vi "Distance + Height to Angle + Length.vi"(2 "Highet [Inch]":dbl, 3 "Distance on ground [Inch]":dbl) -> (0 "Angle [Degrees]":dbl, 1 "Distance[Meter]":dbl)   [LabVIEW 2012]
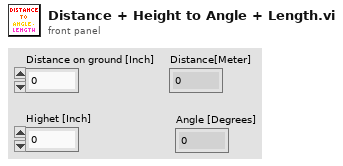
[diagram p1: front panel]
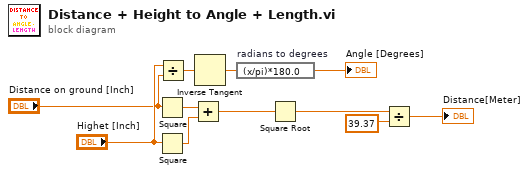
[diagram p0: block diagram]
diagram:
  n1 = Square(x="Distance on ground [Inch]") -> (x^2=w11:dbl)
  n2 = Square(x="Highet [Inch]") -> (x^2=w10:dbl)
  n3 = Divide(x="Highet [Inch]", y="Distance on ground [Inch]") -> (x/y=w8:dbl)
  n4 = Add(x=w11, y=w10) -> (x+y=w9:dbl)
  n5 = Inverse Tangent(1:w8) -> (0:w6:dbl)
  n6 = expression code="(x/pi)*180.0" "radians to degrees"(w6) -> (→"Angle [Degrees]":dbl)
  n7 = Square Root(x=w9) -> (sqrt(x)=w3:dbl)
  n8 = Divide(x=w3, y=39.37) -> (x/y=→"Distance[Meter]":dbl)
